vi "RT Main.vi"() -> ()   [LabVIEW 2019]
uses:
  <vilib>/Platform/TimedLoop/XDataNode/XDataNode.xnode
  <vilib>/Platform/TimedLoop/XDataNode/nitl_modes.ctl
  <vilib>/Platform/TimedLoop/XDataNode/XDNodeRunTimeDep.lvlib
  <vilib>/Platform/TimedLoop/XDataNode/wakeup.ctl
  <vilib>/Platform/TimedLoop/XDataNode/timing_clust.ctl
panel:
  in  "Tab Control":enum32{"Manual", "PID Control"}(tab)
  out "IMU Data":dbl[](graph)
  in  "manual":bool caption="Manual Motor Control"
  in  "Rear Input":dbl min=-1.0 max=1.0 format="%.2f"
  in  "Left Input":dbl min=-1.0 max=1.0 format="%.2f"
  in  "Right Input":dbl min=-1.0 max=1.0 format="%.2f"
  out "Ping Data":dbl[](graph)
  out "Roll PID":dbl[](graph)
  out "Depth PID":dbl[](graph)
  in  "PID":T1
  out "End?":bool
  out "connected?":bool
  out "error out":errorcluster
  in  "stop":bool
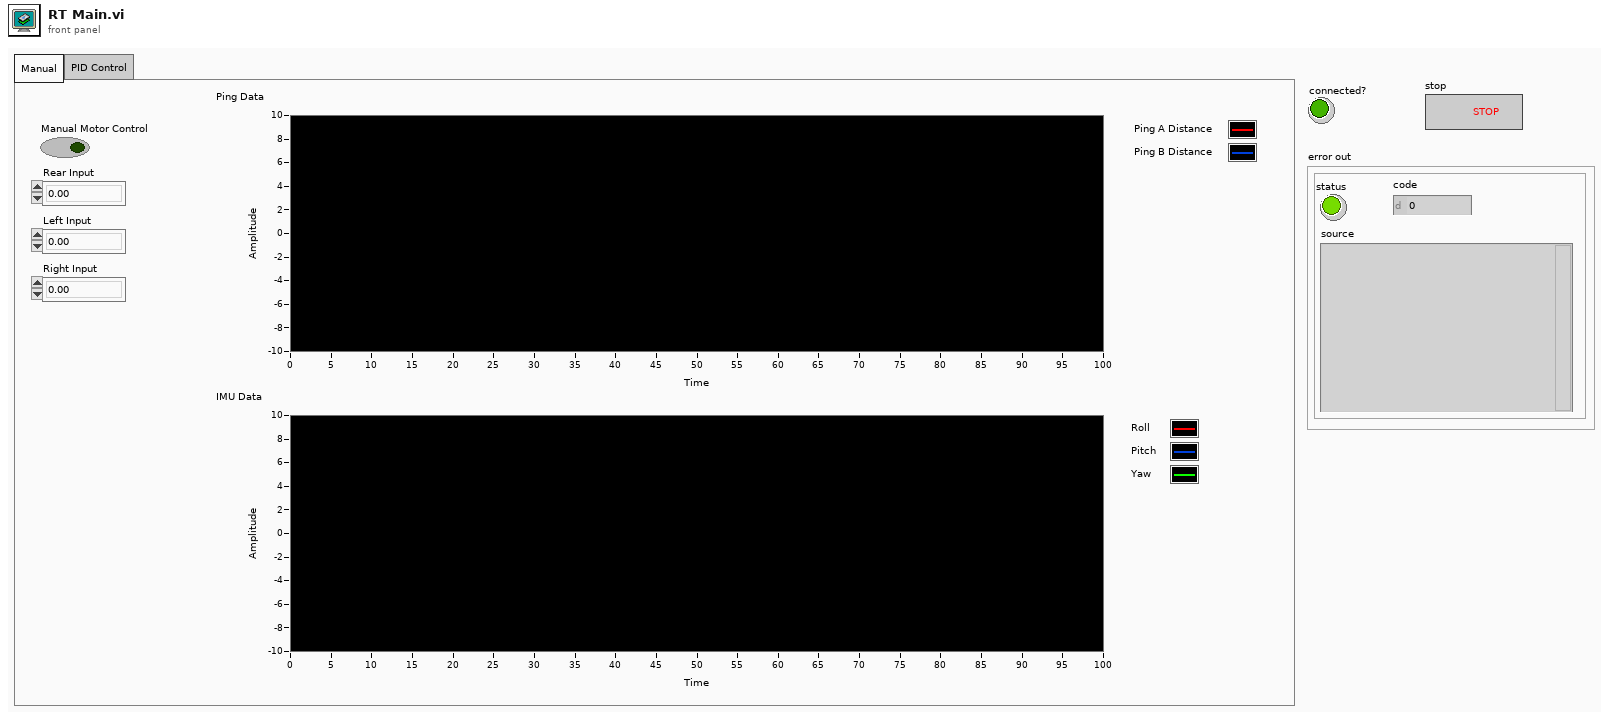
[diagram p1: front panel]
types:
  T1 = cluster{"reinitialize?":bool, "Depth":cluster{"setpoint":dbl, "Gains":cluster{"proportional gain (Kc)":dbl, "integral time (Ti, min)":dbl, "derivative time (Td, min)":dbl}}, "Roll":cluster{"setpoint":dbl, "Gains":cluster{"proportional gain (Kc)":dbl, "integral time (Ti, min)":dbl, "derivative time (Td, min)":dbl}}}
  T2 = typedef "XDNodeRunTimeDep.lvlib/timing_clust.ctl" = cluster{"Expected End [f-1]":u64, "Actual End [f-1]":u64, "Finished Late? [f-1]":bool, "Expected End [i-1]":u64, "Actual End [i-1]":u64, "Finished Late? [i-1]":bool, "Expected Start [i]":u64, "Actual Start [i]":u64, "Expected Start [f]":u64, "Actual Start [f]":u64, "Source Name":string, "Structure Name":string, "Period":i64, "Deadline":i64, "Offset":i64, "Start":i64, "Priority":i32, "Timeout":i32, "Mode":T3, "Wakeup Reason":T4, "Error":errorcluster, "Source Type":string, "Secondary Source Type":string, "Global End Time":u64, "Global Start Time":u64, "Frame Duration":u64, "Iteration Duration":u64, "Assigned CPU":i32, "I/O Scan Engine Mode":u32}
  T3 = typedef "XDNodeRunTimeDep.lvlib/nitl_modes.ctl" = enum32{"No Change", "Process missed periods, maintain original phase", "Discard missed periods, maintain original phase", "Process missed periods, ignore original phase", "Discard missed periods, ignore original phase"}
  T4 = typedef "XDNodeRunTimeDep.lvlib/wakeup.ctl" = enum32{"Normal", "Aborted", "Asynchronous wakeup", "Timing source error", "Timed loop error", "Timeout"}
  T5 = typedef "ROVcluster.ctl" = cluster{"Connections":T6, "sensorData":T7, "outputData":T8, "Writer":cluster{"endpoint":refnum<k21>, "error":errorcluster}, "PID":cluster{"reinitialize?":bool, "Depth":cluster{"setpoint":dbl, "Gains":cluster{"proportional gain (Kc)":dbl, "integral time (Ti, min)":dbl, "derivative time (Td, min)":dbl}}, "Roll":cluster{"setpoint":dbl, "Gains":cluster{"proportional gain (Kc)":dbl, "integral time (Ti, min)":dbl, "derivative time (Td, min)":dbl}}}}
  T6 = typedef "Connections.ctl" = cluster{"Ping1D - A":cluster{"Connection":refnum<visa-resource-name>, "error":errorcluster, "Distance":dbl, "FIFO":cluster{"rt fifo":refnum<k33>, "error":errorcluster}}, "Ping1D - B":cluster{"Connection":refnum<visa-resource-name>, "error":errorcluster, "Distance":dbl, "FIFO":cluster{"rt fifo":refnum<k33>, "error":errorcluster}}, "IMU":cluster{"Error":errorcluster, "FIFO":cluster{"fifo":refnum<k33>, "error":errorcluster}}, "MotorControl":cluster{"Rear":cluster{"Error PWM":errorcluster, "Error Direction":errorcluster}, "Left":cluster{"Error PWM":errorcluster, "Error Direction":errorcluster}, "Right":cluster{"Error PWM":errorcluster, "Error Direction":errorcluster}}}
  T7 = typedef "ROVsensorData.ctl" = cluster{"IMU Data":cluster{"X-Axis":dbl, "Y-Axis":dbl, "Z-Axis":dbl}}
  T8 = typedef "ROVdataOut.ctl" = cluster{"Rotation Angle":dbl, "Rotation Vector":cluster{"x":dbl, "y":dbl, "z":dbl}, "PING A distance":dbl, "Ping B distance":dbl, "angles":cluster{"roll":dbl, "pitch":dbl, "yaw":dbl}}
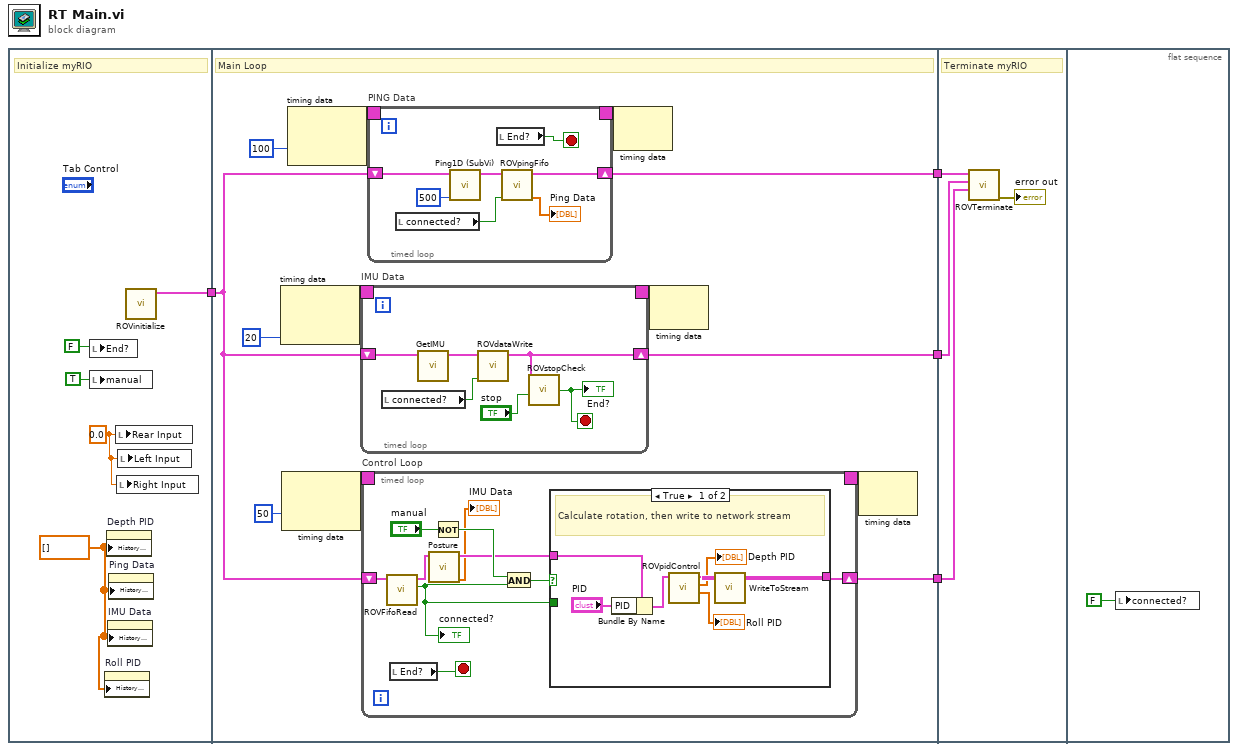
[diagram p0: block diagram]
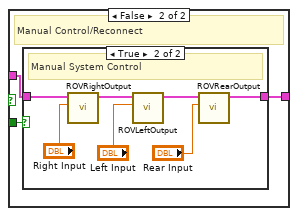
[diagram p2: hidden frame]
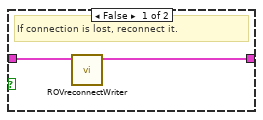
[diagram p3: hidden frame]
diagram:
  n1 = flat-sequence {
    tunnel: [w9] -> w4
    tunnel: w4 -> [w14]
    tunnel: [w19] -> w3
    tunnel: [w18] -> w2
    tunnel: [w10] -> w1
    tunnel: w3 -> [w84]
    tunnel: w2 -> [w85]
    tunnel: w1 -> [w83]
    frame #0 {
      w5 = dbl[] [] ("History Data")
      w6 = 0.0 ("Rear Input")
      # "Initialize myRIO"
      n2 = local write "End?"(FALSE) -> ()
      n3 = local write "manual"(TRUE ("manual")) -> ()
      n4 = property on="Roll PID" class="WFChart (strict)"("History Data"=w5) -> ()  [unwired: 2 in, 2 out]
      n5 = property on="Depth PID" class="WFChart (strict)"("History Data"=w5) -> ()  [unwired: 2 in, 2 out]
      n6 = property on="IMU Data" class="WFChart (strict)"("History Data"=w5) -> ()  [unwired: 2 in, 2 out]
      n7 = property on="Ping Data" class="WFChart (strict)"("History Data"=w5) -> ()  [unwired: 2 in, 2 out]
      n8 = local write "Rear Input"(w6) -> ()
      n9 = local write "Right Input"(w6) -> ()
      n10 = local write "Left Input"(w6) -> ()
      n11 = call "ROVinitialize.vi"() -> ("Cluster out"=w9:T5)  [unwired: 11 in]
    }
    frame #1 {
      # "Main Loop"
      n12 = node-c288(i64 20 ("Period")) -> (w22:T2)  [unwired: 1 in]
      n13 = node-c288(i64 50 ("Period")) -> (w13:T2)  [unwired: 1 in]
      n14 = node-c288(i64 100 ("Period")) -> (w17:T2)  [unwired: 1 in]
      n15 = timed-loop "IMU Data" {
        timing: w22 -> [_]
        timing-out: [_] -> w21
        shift-right: [w73] -> w19
        shift-left: w14 -> [w76]
        stop <- w72 stop-if-true
        n16 = local read "connected?"() -> (w71:bool)
        n17 = call "GetIMU.vi"("Cluster"=w76) -> ("Cluster out"=w75:T5)  [unwired: 10 in]
        n18 = call "ROVdataWrite.vi"("connected?"=w71, "Cluster in"=w75) -> ("Cluster out"=w73:T5)  [unwired: 9 in]
        n19 = call "ROVstopCheck.vi"("stop"="stop", "Cluster"=w73) -> ("stop"=w72:bool)  [unwired: 2 in]
        "End?" <- w72
      }
      n20 = timed-loop "Control Loop" {
        shift-right: [w31] -> w18
        shift-left: w14 -> [w30]
        timing: w13 -> [_]
        timing-out: [_] -> w12
        stop <- w32 stop-if-true
        n21 = call "ROVFifoRead.vi"("Cluster in"=w30) -> ("Connected"=w26:bool, "Cluster out"=w23:T5)  [unwired: 9 in]
        "connected?" <- w26
        n22 = local read "End?"() -> (w32:bool)
        n23 = call "Posture.vi"("Cluster"=w23) -> ("Posture data"=→"IMU Data":dbl[], "Cluster out"=w25:T5)  [unwired: 9 in]
        n24 = Not(x="manual") -> (.not. x?=w28:bool)
        n25 = And(x=w28, y=w26) -> (x .and. y?=w29:bool)
        n26 = case shown="True" w29 {
          tunnel: w25 -> [w36 w42]
          tunnel: [w39 w41] -> w31
          tunnel: w26 -> [_ w40]
          frame True {
            # "Calculate rotation, then write to network stream"
            n27 = Bundle By Name(cluster=w36, "PID"="PID") -> (w35:T5)
            n28 = call "ROVpidControl.vi"("Cluster"=w35) -> ("Roll Array"=→"Roll PID":dbl[], "Depth Array"=→"Depth PID":dbl[], "output cluster"=w38:T5)  [unwired: 8 in]
            n29 = call "WriteToStream.vi"("Cluster"=w38) -> ("output cluster"=w39:T5)  [unwired: 10 in]
          }
          frame False {
            # "Manual Control/Reconnect"
            n30 = case shown="True" w40 {
              tunnel: w42 -> [w44 w51]
              tunnel: [w43 w48] -> w41
              frame False {
                # "If connection is lost, reconnect it."
                n31 = call "ROVreconnectWriter.vi"("Cluster in"=w44) -> ("Cluster out"=w43:T5)  [unwired: 10 in]
              }
              frame True {
                # "Manual System Control"
                n32 = call "ROVRightOutput.vi"("Depth Input"="Right Input", "Cluster"=w51) -> ("output cluster"=w50:T5)  [unwired: 7 in, 2 out]
                n33 = call "ROVLeftOutput.vi"("Depth Input"="Left Input", "Cluster"=w50) -> ("output cluster"=w49:T5)  [unwired: 7 in, 2 out]
                n34 = call "ROVRearOutput.vi"("input"="Rear Input", "Cluster"=w49) -> ("output cluster"=w48:T5)  [unwired: 7 in, 2 out]
              }
            }
          }
        }
      }
      n35 = timed-loop "PING Data" {
        timing: w17 -> [_]
        timing-out: [_] -> w16
        shift-right: [w61] -> w10
        shift-left: w14 -> [w58]
        stop <- w64 stop-if-true
        n36 = local read "connected?"() -> (w60:bool)
        n37 = call "Ping1D (SubVi).vi"("Comm. Delay"=u32 500, "Cluster"=w58) -> ("Cluster out"=w62:T5)  [unwired: 9 in]
        n38 = local read "End?"() -> (w64:bool)
        n39 = call "ROVpingFifo.vi"("connected?"=w60, "Cluster in"=w62) -> ("data Array"=→"Ping Data":dbl[], "Cluster out"=w61:T5)  [unwired: 8 in]
      }
      n40 = node-c288(w16) -> ()  [unwired: 1 out]
      n41 = node-c288(w21) -> ()  [unwired: 1 out]
      n42 = node-c288(w12) -> ()  [unwired: 1 out]
    }
    frame #2 {
      # "Terminate myRIO"
      n43 = call "ROVTerminate.vi"("Cluster in Control"=w85, "Cluster in IMU"=w84, "Cluster in Ping"=w83) -> ("error out"=→"error out":errorcluster)  [unwired: 8 in]
    }
    frame #3 {
      n44 = local write "connected?"(FALSE) -> ()
    }
  }
